vi "check-instruction.vi"(0 "instruction":i32[](array[numeric]), 1 "car X":dbl, 2 "Car Y":dbl, 3 "scale":dbl, 4 "start time":u32) -> (5 "complete":bool)   [LabVIEW 2015]
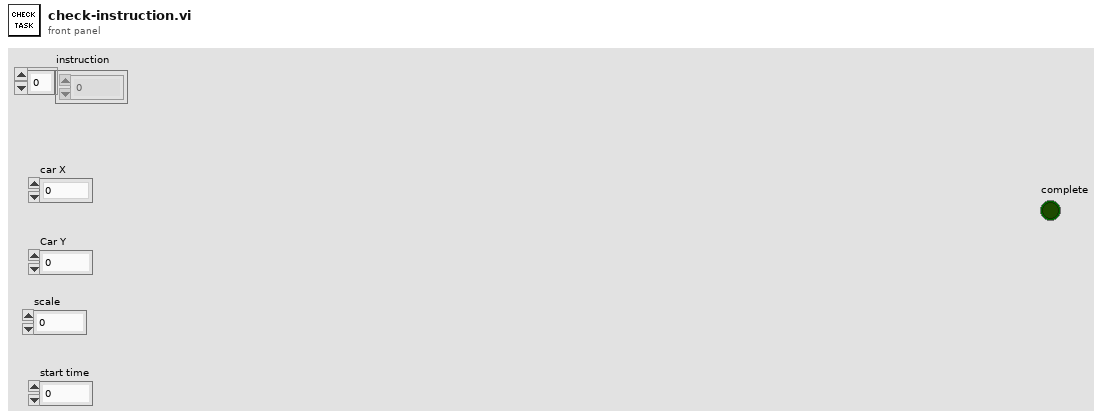
[diagram p1: front panel]
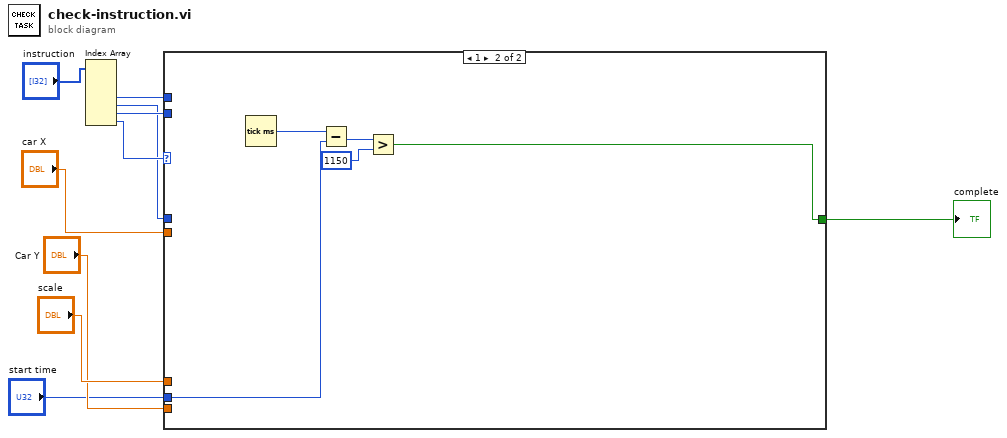
[diagram p0: block diagram]
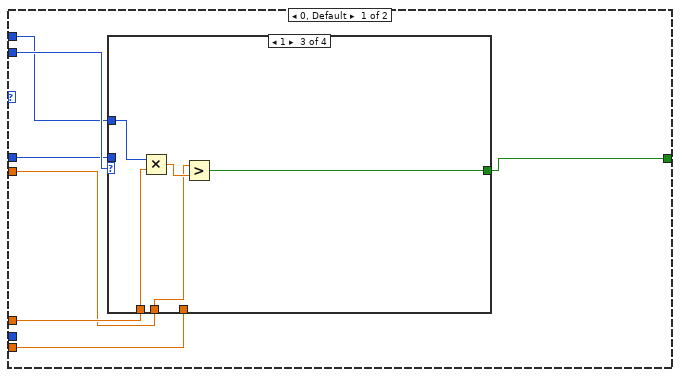
[diagram p2: hidden frame]
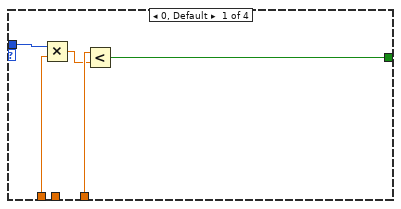
[diagram p3: hidden frame]
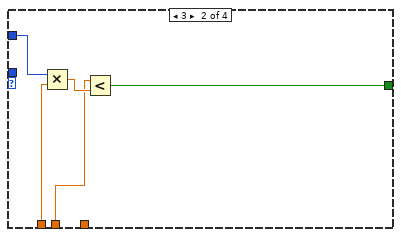
[diagram p4: hidden frame]
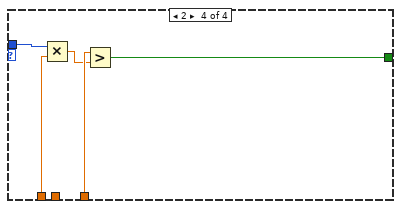
[diagram p5: hidden frame]
diagram:
  n1 = Index Array(array="instruction") -> (element #3=w4:i32, element #4=w5:i32, element #5=w8:i32, element #6=w9:i32)  [unwired: 6 in, 2 out]
  n2 = case shown="1" w9 {
    tunnel: w8 -> [w17 _]
    tunnel: [w16 w38] -> w7
    tunnel: "scale" -> [w15 _]
    tunnel: w5 -> [w14 _]
    tunnel: w4 -> [w13 _]
    tunnel: "Car Y" -> [w12 _]
    tunnel: "car X" -> [w11 _]
    tunnel: "start time" -> [_ w41]
    frame 0, Default {
      n3 = case shown="1" w17 {
        tunnel: w12 -> [w22 _ _ w37]
        tunnel: w15 -> [w20 w26 w31 w35]
        tunnel: w14 -> [w19 _ _ w34]
        tunnel: [w18 w25 w30 w33] -> w16
        tunnel: w13 -> [_ w24 w29 _]
        tunnel: w11 -> [_ w23 w28 _]
        frame 0, Default {
          n4 = Multiply(x=w19, y=w20) -> (x*y=w21:dbl)
          n5 = Less?(x=w22, y=w21) -> (x < y?=w18:bool)
        }
        frame 3 {
          n6 = Multiply(x=w24, y=w26) -> (x*y=w27:dbl)
          n7 = Less?(x=w23, y=w27) -> (x < y?=w25:bool)
        }
        frame 1 {
          n8 = Multiply(x=w29, y=w31) -> (x*y=w32:dbl)
          n9 = Greater?(x=w28, y=w32) -> (0:w30:bool)
        }
        frame 2 {
          n10 = Multiply(x=w34, y=w35) -> (x*y=w36:dbl)
          n11 = Greater?(x=w37, y=w36) -> (0:w33:bool)
        }
      }
    }
    frame 1 {
      n12 = Tick Count (ms)() -> (millisecond timer value=w42:u32)
      n13 = Subtract(x=w42, y=w41) -> (x-y=w40:u32)
      n14 = Greater?(x=w40, y=1150) -> (0:w38:bool)
    }
  }
  "complete" <- w7
